vi "Instrument Type ID.vi"() -> (1 "instrument type id":string="niScope")   [LabVIEW 2020, in "NI Session Management niScope.lvlib"]
uses:
  NI Session Management niScope.lvlib
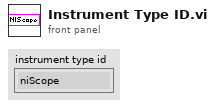
[diagram p1: front panel]
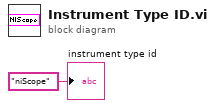
[diagram p0: block diagram]
diagram:
  "instrument type id" <- "niScope" ("instrument type id")
